vi "WriteSignalToTXT_TU.vi"() -> ()   [LabVIEW 2025]
panel:
  out "file path out":path
  out "error out":errorcluster
  in  "file path in":path
  in  "signal in":waveform(dbl)
  in  "error in":errorcluster
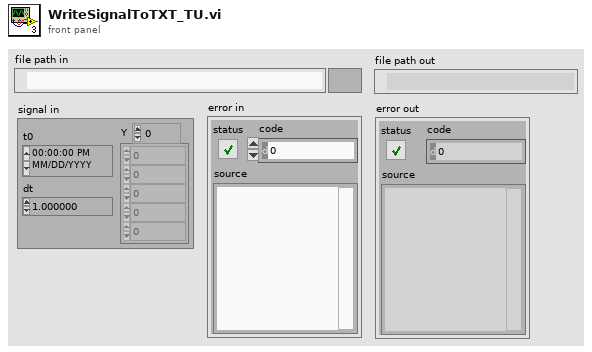
[diagram p1: front panel]
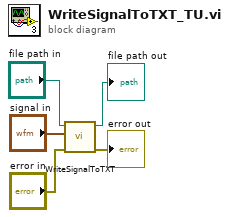
[diagram p0: block diagram]
diagram:
  n1 = call "WriteSignalToTXT.vi"("error in"="error in", "signal in"="signal in", "file path in"="file path in") -> ("error out"=→"error out":errorcluster, "file path out"=→"file path out":path)  [unwired: 7 in]
